vi "WalkThroughExample.vi"() -> ()   [LabVIEW 2019]
uses:
  <vilib>/Rock Robotics/WPI/ThirdParty/JAS_Junk/TrajLib/LINEAR_SYSTEM.ctl
  <vilib>/Analysis/Matrix/Datatypes/RealMatrix.ctl
  <vilib>/Rock Robotics/WPI/ThirdParty/JAS_Junk/TrajLib/DCMOTOR.CTL
  <vilib>/Rock Robotics/WPI/ThirdParty/JAS_Junk/TrajLib/LINEAR_QUADRATIC_REGULATOR.ctl
  <vilib>/Rock Robotics/WPI/ThirdParty/JAS_Junk/TrajLib/KALMAN_FILTER.ctl
  <vilib>/Rock Robotics/WPI/ThirdParty/JAS_Junk/TrajLib/LINEAR_SYSTEM_LOOP.ctl
  <vilib>/Rock Robotics/WPI/ThirdParty/JAS_Junk/TrajLib/LINEAR_PLANT_INV_FF.ctl
  <vilib>/Rock Robotics/WPI/ThirdParty/JAS_Junk/TrajLib/FLYWHEEL_SIM.ctl
  <vilib>/Rock Robotics/WPI/ThirdParty/JAS_Junk/TrajLib/LINEAR_SYSTEM_SIM.ctl
  <vilib>/numeric/Random Number (Range) DBL.vi
  <vilib>/Rock Robotics/WPI/ThirdParty/JAS_Junk/TrajLib/DCMotor_New.vi
  <vilib>/Rock Robotics/WPI/ThirdParty/JAS_Junk/TrajLib/MatBuilder_Create.vi
  <vilib>/Rock Robotics/WPI/ThirdParty/JAS_Junk/TrajLib/MatrixHelper_Zero.vi
  <vilib>/Rock Robotics/WPI/ThirdParty/JAS_Junk/TrajLib/MatBuilder_Fill.vi
  <vilib>/Rock Robotics/WPI/ThirdParty/JAS_Junk/TrajLib/Matrix_Ident.vi
  <vilib>/Rock Robotics/WPI/ThirdParty/JAS_Junk/TrajLib/LinearSystem_New.vi
  <vilib>/Analysis/7linalg.llb/Create Special Matrix.vi
  <vilib>/Analysis/7linalg.llb/Create Special Real Matrix.vi
  <vilib>/Rock Robotics/WPI/ThirdParty/JAS_Junk/TrajLib/Trajectory_Library.lvlib
  <vilib>/Analysis/Matrix/NI_Matrix.lvlib
panel:
  in  "Tab Control":T1(tab)
  out "m_flywheelPlant":T2
  out "Shooter Motor":T4 {"Jr_KgM2" format="%13.5p"; "L_H" format="%13.5p"; "Kt_NMPerAmp" format="%13.5p"; "KvINV_RadPerSecPerVolt" format="%13.5p"; "R_Ohms" format="%13.5p"; "FreeSpeed_RadPerSec" format="%13.5p"; "FreeCurrent_Amps" format="%13.5p"; "StallCurrent_Amps" format="%13.5p"; "StallTorque_NM" format="%13.5p"; "nominalVoltage_Volts" format="%13.5p"}
  out "m_flywheelPlant_ALT":T2
  out "KalmanFilter":T5
  out "Kalman Error":bool
  out "LinearQuadraticRegulator":T6
  out "LQR Error":bool
  out "Linear System Loop":T7
  out "LinSysLoop_Error":bool
  out "m_FlyWheelSim":T9 {"GearBox"."Jr_KgM2" format="%13.5p"; "GearBox"."L_H" format="%13.5p"; "GearBox"."Kt_NMPerAmp" format="%13.5p"; "GearBox"."KvINV_RadPerSecPerVolt" format="%13.5p"; "GearBox"."R_Ohms" format="%13.5p"; "GearBox"."FreeSpeed_RadPerSec" format="%13.5p"; "GearBox"."FreeCurrent_Amps" format="%13.5p"; "GearBox"."StallCurrent_Amps" format="%13.5p"; "GearBox"."StallTorque_NM" format="%13.5p"; "GearBox"."nominalVoltage_Volts" format="%13.5p"}
  out "Shooting A":T3
  out "Shooting B":T3
  out "Battery Voltage":dbl format="%20.3f"
  in  "Shoot ball":bool
  out "CO Chart":cluster{dbl, "Voltage":dbl}(graph)
  in  "Shooter On/Off":bool
  out "Encoer Speed\nRad/Sec":dbl(slide) scale=0.0..300.0
  out "Speed":dbl format="%20.3f"
  out "Cor Err":bool
  out "Kalman Filtered\nSpeed":dbl format="%20.3f"
  out "PV Chart":T11(graph)
  out "Predict Err":bool
  out "Motor Volt Dmd (CO)":dbl format="%20.3f"
  out "shoot":bool
  out "Shoot Done":bool
  # "<States,States>"
  # "<States,Inputs>"
  # "<Outputs,States>"
  # "<Outputs,Inputs>"
  # "<States,States>"
  # "<States,Inputs>"
  # "<Outputs,States>"
  # "<Outputs,Inputs>"
  # "Steady State Gain  \n<States,Outputs>"
  # "State Estimate <Statess,1>"
  # "<States,States>"
  # "<States,Inputs>"
  # "<Outputs,States>"
  # "<Outputs,Inputs>"
  # "Ref State <States,1>"
  # "Comp and capped \noutput <Inputs,1>"
  # "Controller gain\n<Inputs,States>"
  # "<States,1>"
  # "<FUTURE --- CLAMP TYPE -- For now\nuse Normalize>"
  # "Steady State Gain  \n<States,Outputs>"
  # "State Estimate <Statess,1>"
  # "<States,States>"
  # "<States,Inputs>"
  # "<Outputs,States>"
  # "<Outputs,Inputs>"
  # "<States,1>"
  # "<Inputs,1>"
  # "<States,Inputs>"
  # "<States,States>"
  # "Ref State <States,1>"
  # "Comp and capped \noutput <Inputs,1>"
  # "Controller gain\n<Inputs,States>"
  # "<States, 1>"
  # "<Outputs, 1>"
  # "<Inputs, 1>"
  # "<Outputs, 1>"
  # "<States,States>"
  # "<States,Inputs>"
  # "<Outputs,States>"
  # "<Outputs,Inputs>"
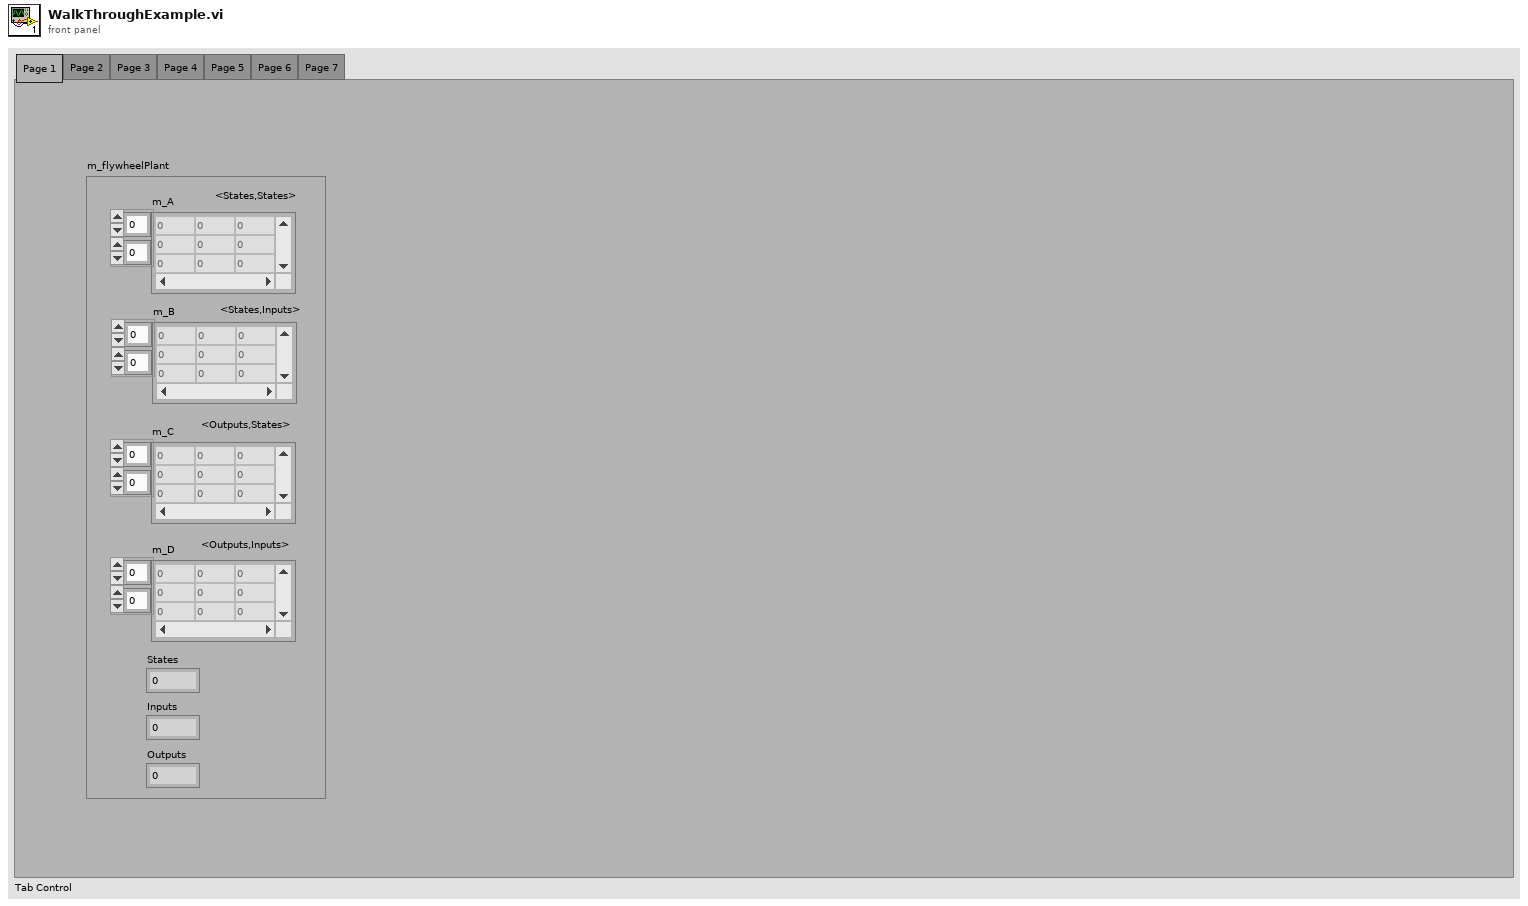
[diagram p1: front panel]
types:
  T1 = enum32{"Page 1", "Page 2", "Page 3", "Page 4", "Page 5", "Page 6", "Page 7"}
  T2 = typedef "Trajectory_Library.lvlib/LINEAR_SYSTEM.ctl" = cluster{"m_A":T3, "m_B":T3, "m_C":T3, "m_D":T3, "States":i32, "Inputs":i32, "Outputs":i32}
  T3 = typedef "NI_Matrix.lvlib/RealMatrix.ctl" = dbl[][]
  T4 = typedef "Trajectory_Library.lvlib/DCMOTOR.CTL" = cluster{"nominalVoltage_Volts":dbl, "StallTorque_NM":dbl, "StallCurrent_Amps":dbl, "FreeCurrent_Amps":dbl, "FreeSpeed_RadPerSec":dbl, "R_Ohms":dbl, "KvINV_RadPerSecPerVolt":dbl, "Kt_NMPerAmp":dbl, "L_H":dbl, "Jr_KgM2":dbl}
  T5 = typedef "Trajectory_Library.lvlib/KALMAN_FILTER.ctl" = cluster{"m_K":T3, "m_xHat":T3, "States":i32, "Outputs":i32, "m_Plant":T2}
  T6 = typedef "Trajectory_Library.lvlib/LINEAR_QUADRATIC_REGULATOR.ctl" = cluster{"m_r":T3, "m_U":T3, "m_K":T3, "States":i32, "Inputs":i32}
  T7 = typedef "Trajectory_Library.lvlib/LINEAR_SYSTEM_LOOP.ctl" = cluster{"Controller":T6, "FeedForward":T8, "Observer":T5, "Next_R":T3, "Clamp Max":T3}
  T8 = typedef "Trajectory_Library.lvlib/LINEAR_PLANT_INV_FF.ctl" = cluster{"m_R":T3, "m_Uff":T3, "m_B":T3, "m_A":T3, "States":i32, "Inputs":i32}
  T9 = typedef "Trajectory_Library.lvlib/FLYWHEEL_SIM.ctl" = cluster{"LinearSystemSim":T10, "GearBox":T4, "Gearing":dbl}
  T10 = typedef "Trajectory_Library.lvlib/LINEAR_SYSTEM_SIM.ctl" = cluster{"m_Plant":T2, "m_X":T3, "m_Y":T3, "m_U":T3, "MeasureStdDev":T3}
  T11 = cluster{"upper limit":dbl, "Real Matrix Element":dbl, "Real Matrix Element":dbl}
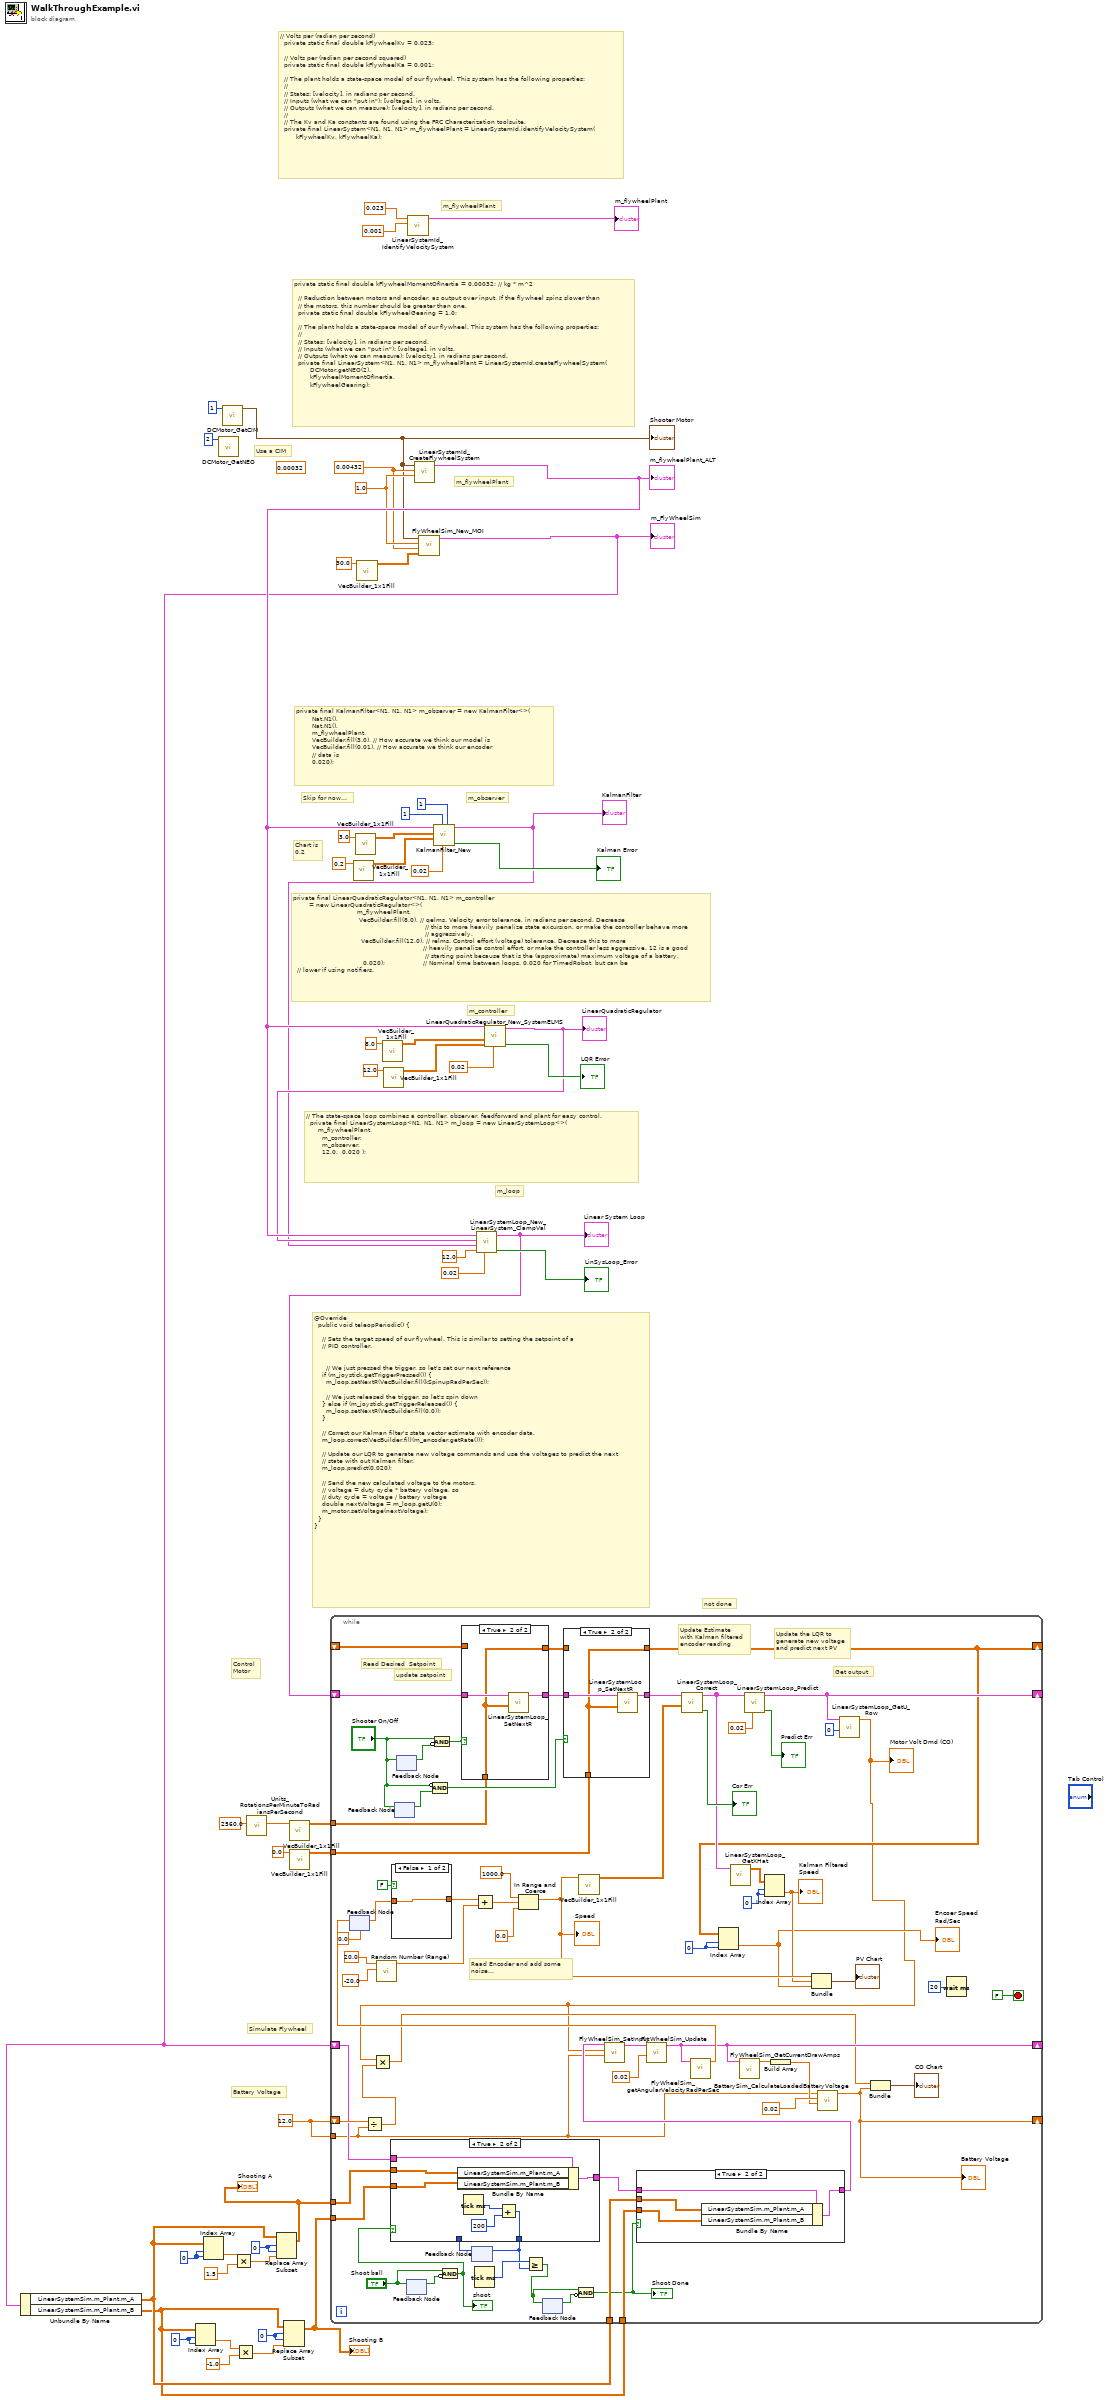
[diagram p0: block diagram]
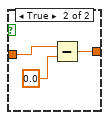
[diagram p4: hidden frame]
diagram:
  w11 = 0 ("index (row)")
  w12 = 0 ("index (row)")
  w13 = 0 ("index (row)")
  w14 = 0 ("index (row)")
  w18 = 12.0
  w19 = 0.00432 ("jKgMetersSquared")
  w22 = 1.0 ("G")
  (unwired) 0.00032 ("jKgMetersSquared")
  # "Control\nMotor"
  # "Simulate Flywheel"
  # "Use a CIM"
  # "Battery Voltage"
  # "Chart is\n0.2"
  # "Skip for now..."
  # "m_loop"
  # "m_controller"
  # "m_observer"
  # "not done"
  # "@Override\n  public void teleopPeriodic() {\n\n    // Sets the target speed of our flywheel. This is similar to setting the setpoint of a\n    // PID controller.\n\n\n      // We just pressed the trigger, so let's set our next reference\n    if (m_joystick.getTriggerPressed()) {\n      m_loop.setNextR(VecBuilder.fill(kSpinupRadPerSec));\n\n      // We just released the trigger, so let's spin down\n    } else if (m_joystick.getTriggerReleased()) {\n      m_loop.setNextR(VecBuilder.fill(0.0));\n    }\n\n    // Correct our Kalman filter's state vector estimate with encoder data.\n    m_loop.correct(VecBuilder.fill(m_encoder.getRate()));\n\n    // Update our LQR to generate new voltage commands and use the voltages to predict the next\n    // state with out Kalman filter.\n    m_loop.predict(0.020);\n\n    // Send the new calculated voltage to the motors.\n    // voltage = duty cycle * battery voltage, so\n    // duty cycle = voltage / battery voltage\n    double nextVoltage = m_loop.getU(0);\n    m_motor.setVoltage(nextVoltage);\n  }\n}"
  # "// The state-space loop combines a controller, observer, feedforward and plant for easy control.\n  private final LinearSystemLoop<N1, N1, N1> m_loop = new LinearSystemLoop<>(\n      m_flywheelPlant,\n        m_controller,\n        m_observer,\n        12.0,  0.020 );"
  # "private final LinearQuadraticRegulator<N1, N1, N1> m_controller\n        = new LinearQuadraticRegulator<>(\n                                m_flywheelPlant,\n                                 VecBuilder.fill(8.0), // qelms. Velocity error tolerance, in radians per second. Decrease\n                                                                  // this to more heavily penalize state excursion, or make the controller behave more\n                                                                  // aggressively.\n                                  VecBuilder.fill(12.0), // relms. Control effort (voltage) tolerance. Decrease this to more\n                                                                 // heavily penalize control effort, or make the controller less aggressive. 12 is a good\n                                                                  // starting point because that is the (approximate) maximum voltage of a battery.\n                                   0.020);                   // Nominal time between loops. 0.020 for TimedRobot, but can be\n  // lower if using notifiers."
  # "private final KalmanFilter<N1, N1, N1> m_observer = new KalmanFilter<>(\n        Nat.N1(), \n        Nat.N1(),\n        m_flywheelPlant,\n        VecBuilder.fill(3.0), // How accurate we think our model is\n        VecBuilder.fill(0.01), // How accurate we think our encoder\n        // data is\n        0.020);"
  # "m_flywheelPlant"
  # "private static final double kFlywheelMomentOfInertia = 0.00032; // kg * m^2\n\n  // Reduction between motors and encoder, as output over input. If the flywheel spins slower than\n  // the motors, this number should be greater than one.\n  private static final double kFlywheelGearing = 1.0;\n\n  // The plant holds a state-space model of our flywheel. This system has the following properties:\n  //\n  // States: [velocity], in radians per second.\n  // Inputs (what we can \"put in\"): [voltage], in volts.\n  // Outputs (what we can measure): [velocity], in radians per second.\n  private final LinearSystem<N1, N1, N1> m_flywheelPlant = LinearSystemId.createFlywheelSystem(\n        DCMotor.getNEO(2),\n        kFlywheelMomentOfInertia,\n        kFlywheelGearing);"
  # "m_flywheelPlant"
  # "// Volts per (radian per second)\n  private static final double kFlywheelKv = 0.023;\n\n  // Volts per (radian per second squared)\n  private static final double kFlywheelKa = 0.001;\n\n  // The plant holds a state-space model of our flywheel. This system has the following properties:\n  //\n  // States: [velocity], in radians per second.\n  // Inputs (what we can \"put in\"): [voltage], in volts.\n  // Outputs (what we can measure): [velocity], in radians per second.\n  //\n  // The Kv and Ka constants are found using the FRC Characterization toolsuite.\n  private final LinearSystem<N1, N1, N1> m_flywheelPlant = LinearSystemId.identifyVelocitySystem(\n        kFlywheelKv, kFlywheelKa);"
  n1 = call <vilib>:"DCMotor_GetNEO.vi"("Num Motors"=2) -> ()  [unwired: 10 in, 1 out]
  n2 = call <vilib>:"DCMotor_GetCIM.vi"("Num Motors"=1) -> ("DCMOTOR"=w17:T4)  [unwired: 10 in]
  "Shooter Motor" <- w17
  n3 = call <vilib>:"Units_RotationsPerMinuteToRadiansPerSecond.vi"("RotationsPerMinute"=2560.0) -> ("RadiansPerSecond"=w26:dbl)  [unwired: 10 in]
  n4 = call <vilib>:"VecBuilder_1x1Fill.vi"("R0_C0"=w26) -> ("output matrix"=w24:T3)  [unwired: 10 in]
  n5 = call <vilib>:"VecBuilder_1x1Fill.vi"("R0_C0"=0.0) -> ("output matrix"=w23:T3)  [unwired: 10 in]
  n6 = call <vilib>:"VecBuilder_1x1Fill.vi"("R0_C0"=0.2) -> ("output matrix"=w36:T3)  [unwired: 10 in]
  n7 = call <vilib>:"VecBuilder_1x1Fill.vi"("R0_C0"=3.0) -> ("output matrix"=w37:T3)  [unwired: 10 in]
  n8 = call <vilib>:"VecBuilder_1x1Fill.vi"("R0_C0"=30.0) -> ("output matrix"=w21:T3)  [unwired: 10 in]
  n9 = call <vilib>:"VecBuilder_1x1Fill.vi"("R0_C0"=8.0) -> ("output matrix"=w45:T3)  [unwired: 10 in]
  n10 = call <vilib>:"VecBuilder_1x1Fill.vi"("R0_C0"=12.0) -> ("output matrix"=w43:T3)  [unwired: 10 in]
  n11 = call <vilib>:"LinearSystemId_IdentifyVelocitySystem.vi"("kA"=0.001, "kV"=0.023) -> ("Linearsystem"=→"m_flywheelPlant":T2)  [unwired: 8 in, 1 out]
  n12 = call <vilib>:"LinearSystemId_CreateFlywheelSystem.vi"("G"=w22, "jKgMetersSquared"=w19, "DCMOTOR"=w17) -> ("Linearsystem"=w34:T2)  [unwired: 7 in, 1 out]
  "m_flywheelPlant_ALT" <- w34
  n13 = call <vilib>:"FlyWheelSim_New_MOI.vi"("MeasurementStdDev"=w21, "jKgMetersSquared"=w19, "Gearing"=w22, "GearBox"=w17) -> ("FlyWheelSim"=w15:T9)  [unwired: 6 in, 1 out]
  "m_FlyWheelSim" <- w15
  n14 = Unbundle By Name(w15) -> ("LinearSystemSim.m_Plant.m_A"=w4:T3, "LinearSystemSim.m_Plant.m_B"=w3:T3)
  n15 = Index Array(array=w3, index (row)=w14, index (col)=w14) -> (element=w6:dbl)
  n16 = Index Array(array=w4, index (row)=w13, index (col)=w13) -> (element=w10:dbl)
  n17 = Multiply(x=w10, y=1.5) -> (x*y=w8:dbl)
  n18 = Multiply(x=w6, y=-1.0) -> (x*y=w5:dbl)
  n19 = Replace Array Subset(array=w4, new element=w8, index (row)=w11, index (col)=w11) -> (w2:T3)
  "Shooting A" <- w2
  n20 = Replace Array Subset(array=w3, new element=w5, index (row)=w12, index (col)=w12) -> (w1:T3)
  "Shooting B" <- w1
  n21 = call <vilib>:"KalmanFilter_New.vi"("States"=1, "dt_Seconds"=0.02, "Outputs"=1, "MeasurementStdDevs"=w36, "StateStdDevs"=w37, "Plant"=w34) -> ("Error"=→"Kalman Error":bool, "KalmanFilter"=w32:T5)  [unwired: 4 in]
  "KalmanFilter" <- w32
  n22 = call <vilib>:"LinearQuadraticRegulator_New_SystemELMS.vi"("dt_Seconds"=0.02, "Relms"=w43, "Qelms"=w45, "LINEARSYSTEM"=w34) -> ("Error"=→"LQR Error":bool, "LinearQuadraticRegulator"=w33:T6)  [unwired: 6 in]
  "LinearQuadraticRegulator" <- w33
  n23 = call <vilib>:"LinearSystemLoop_New_LinearSystem_ClampVal.vi"("dT_Seconds"=0.02, "Max_Voltage"=12.0, "Observer"=w32, "Controller"=w33, "Plant"=w34) -> ("Error"=→"LinSysLoop_Error":bool, "Linear System Loop"=w28:T7)  [unwired: 5 in]
  "Linear System Loop" <- w28
  n24 = while {
    shift-right: [w93] -> _
    shift-left: w28 -> [w114]
    tunnel: w24 -> [w112]
    tunnel: w23 -> [w111]
    shift-right: [w79] -> _
    shift-left: w15 -> [w72]
    shift-right: [w85] -> _
    shift-left: _ -> [w86]
    shift-right: [w74] -> _
    shift-left: w18 -> [w80]
    tunnel: w18 -> [w54]
    tunnel: w4 -> [w65]
    tunnel: w3 -> [w64]
    tunnel: w2 -> [w63]
    tunnel: w1 -> [w62]
    stop <- FALSE stop-if-true
    w84 = 0 ("index (row)")
    w101 = 0 ("index (row)")
    # "Get output"
    # "Update the LQR to \ngenerate new voltage\nand predict next PV"
    # "update setpoint"
    # "Read Desired  Setpoint"
    # "Update Estimate\nwith Kalman filtered\nencoder reading"
    # "Read Encoder and add some \nnoise..."
    n25 = feedback #1(0.0 ("Velocity_RadPerSec")) -> (w82:dbl)
    n26 = Divide(x=w80, y=w54) -> (x/y=w55:dbl)
    n27 = call-poly <vilib>:"Random Number (Range).vi"("lower bound (0)"=-20.0, "upper bound (100)"=20.0) -> ("number"=w108:dbl)  [unwired: 9 in]
    n28 = case shown="False" FALSE {
      tunnel: w82 -> [w136 w139]
      tunnel: [w136 w138] -> w81
      frame False {
      }
      frame True {
        n29 = Subtract(x=w139, y=0.0) -> (x-y=w138:dbl)
      }
    }
    n30 = feedback #2() -> (w118:bool)  [unwired: 1 in]
    n31 = feedback-in #2("Shooter On/Off") -> ()
    n32 = feedback-in #3("Shooter On/Off") -> ()
    n33 = feedback #3() -> (w119:bool)  [unwired: 1 in]
    n34 = feedback-in #4("Shoot ball") -> ()
    n35 = feedback #4() -> (w67:bool)  [unwired: 1 in]
    n36 = Compound Arithmetic op=AND(invert "Shooter On/Off", w118) -> (w115:bool)
    n37 = Compound Arithmetic op=AND("Shooter On/Off", invert w119) -> (w116:bool)
    n38 = Compound Arithmetic op=AND("Shoot ball", invert w67) -> (w66:bool)
    "shoot" <- w66
    n39 = case shown="True" w116 {
      tunnel: w114 -> [w146 w148]
      tunnel: [w146 w149] -> w113
      tunnel: w112 -> [_ w147]
      tunnel: [w145 w147] -> w87
      tunnel: w86 -> [w145 _]
      frame False {
      }
      frame True {
        n40 = call <vilib>:"LinearSystemLoop_SetNextR.vi"("R"=w147, "input inear System Loop"=w148) -> ("out Linear System Loop"=w149:T7)  [unwired: 8 in, 1 out]
      }
    }
    n41 = feedback #5() -> (w56:u32)  [unwired: 1 in]
    n42 = case shown="True" w66 {
      tunnel: w72 -> [w128 w135]
      tunnel: [w128 w132] -> w71
      tunnel: w63 -> [_ w134]
      tunnel: w62 -> [_ w133]
      tunnel: [w127 w129] -> w57
      tunnel: w56 -> [w127 _]
      frame False {
      }
      frame True {
        n43 = Bundle By Name(cluster=w135, "LinearSystemSim.m_Plant.m_A"=w134, "LinearSystemSim.m_Plant.m_B"=w133) -> (w132:T9)
        n44 = Tick Count (ms)() -> (millisecond timer value=w131:u32)
        n45 = Add(x=w131, y=u32 200) -> (x+y=w129:u32)
      }
    }
    n46 = feedback-in #5(w57) -> ()
    n47 = Tick Count (ms)() -> (millisecond timer value=w61:u32)
    n48 = Add(x=w81, y=w108) -> (x+y=w106:dbl)
    n49 = In Range and Coerce(upper limit=1000.0, x=w106, lower limit=0.0) -> (coerced(x)=w99:dbl)  [unwired: 1 out]
    "Speed" <- w99
    n50 = Greater Or Equal?(x=w61, y=w57) -> (x >= y?=w59:bool)
    n51 = feedback #6() -> (w60:bool)  [unwired: 1 in]
    n52 = feedback-in #6(w59) -> ()
    n53 = case shown="True" w115 {
      tunnel: w113 -> [w141 w143]
      tunnel: [w141 w144] -> w104
      tunnel: w111 -> [_ w142]
      tunnel: w87 -> [w140 _]
      tunnel: [w140 w142] -> w85
      frame False {
      }
      frame True {
        n54 = call <vilib>:"LinearSystemLoop_SetNextR.vi"("R"=w142, "input inear System Loop"=w143) -> ("out Linear System Loop"=w144:T7)  [unwired: 8 in, 1 out]
      }
    }
    n55 = Compound Arithmetic op=AND(w59, invert w60) -> (w58:bool)
    "Shoot Done" <- w58
    n56 = call <vilib>:"VecBuilder_1x1Fill.vi"("R0_C0"=w99) -> ("output matrix"=w103:T3)  [unwired: 10 in]
    n57 = case shown="True" w58 {
      tunnel: w71 -> [w122 w126]
      tunnel: [w122 w125] -> w70
      tunnel: w65 -> [_ w124]
      tunnel: w64 -> [_ w123]
      frame False {
      }
      frame True {
        n58 = Bundle By Name(cluster=w126, "LinearSystemSim.m_Plant.m_A"=w124, "LinearSystemSim.m_Plant.m_B"=w123) -> (w125:T9)
      }
    }
    n59 = call <vilib>:"LinearSystemLoop_Correct.vi"("Y"=w103, "input inear System Loop"=w104) -> ("Error"=→"Cor Err":bool, "out Linear System Loop"=w96:T7)  [unwired: 8 in]
    n60 = Index Array(array=w85, index (row)=w84, index (col)=w84) -> (element=w83:dbl)
    "Encoer Speed\nRad/Sec" <- w83
    n61 = call <vilib>:"LinearSystemLoop_GetXHat.vi"("input inear System Loop"=w96) -> ("XHat"=w100:T3)  [unwired: 10 in]
    n62 = call <vilib>:"LinearSystemLoop_Predict.vi"("dT_Seconds"=0.02, "input inear System Loop"=w96) -> ("Error"=→"Predict Err":bool, "out Linear System Loop"=w93:T7)  [unwired: 8 in]
    n63 = Index Array(array=w100, index (row)=w101, index (col)=w101) -> (element=w98:dbl)
    "Kalman Filtered\nSpeed" <- w98
    n64 = Bundle("upper limit"=w99, "Real Matrix Element"=w98, "Real Matrix Element"=w83) -> (→"PV Chart":T11)  [unwired: 1 in]
    n65 = call <vilib>:"LinearSystemLoop_GetU_Row.vi"("Row"=0, "input inear System Loop"=w93) -> ("U"=w53:dbl)  [unwired: 9 in]
    "Motor Volt Dmd (CO)" <- w53
    n66 = Multiply(x=w53, y=w55) -> (x*y=w73:dbl)
    n67 = call <vilib>:"FlyWheelSim_SetInput.vi"("Battery_Volts"=w54, "Volts"=w53, "FlyWheelSim"=w70) -> ("out FlyWheelSim"=w91:T9)  [unwired: 8 in]
    n68 = call <vilib>:"FlyWheelSim_Update.vi"("dT_Seconds"=0.02, "FlyWheelSim"=w91) -> ("out FlyWheelSim"=w79:T9)  [unwired: 8 in, 1 out]
    n69 = call <vilib>:"FlyWheelSim_getAngularVelocityRadPerSec.vi"("FlyWheelSim"=w79) -> ("Velocity_RadPerSec"=w89:dbl)  [unwired: 10 in]
    n70 = feedback-in #1(w89) -> ()
    n71 = call <vilib>:"FlyWheelSim_GetCurrentDrawAmps.vi"("FlyWheelSim"=w79) -> ("Current_Amps"=w77:dbl)  [unwired: 10 in]
    n72 = Build Array(w77) -> (w76:dbl[])
    n73 = call <vilib>:"BatterySim_CalculateLoadedBatteryVoltage.vi"("Currents"=w76, "Resistance_Ohms"=0.02, "NominalVoltage"=w54) -> ("Voltage"=w74:dbl)  [unwired: 8 in]
    "Battery Voltage" <- w74
    n74 = Bundle(w73, "Voltage"=w74) -> (→"CO Chart":cluster{dbl, "Voltage":dbl})  [unwired: 1 in]
    n75 = Wait (ms)(milliseconds to wait=u32 20) -> ()  [unwired: 1 out]
  }
